vi "Start Plugin.vi"(8 "error in (no error)":errorcluster, 11 "Plugin in":refnum<class "Plugin.lvclass">) -> (0 "error out":errorcluster, 3 "Plugin out":refnum<class "Plugin.lvclass">)   [LabVIEW 2019, in "DSF Core.lvlib" / "Plugin.lvclass"]
uses:
  Plugin.lvclass
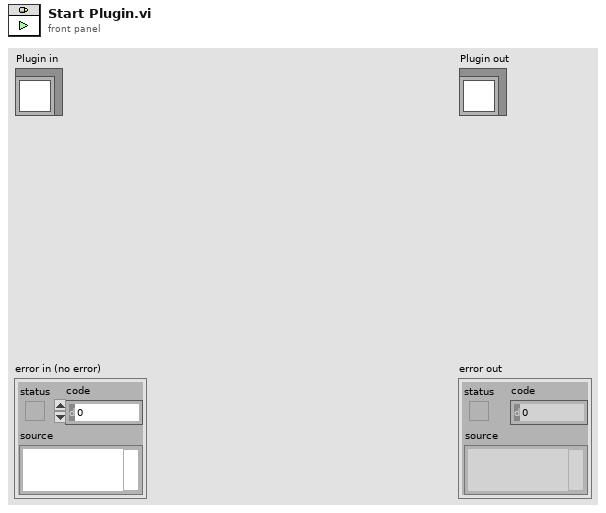
[diagram p1: front panel]
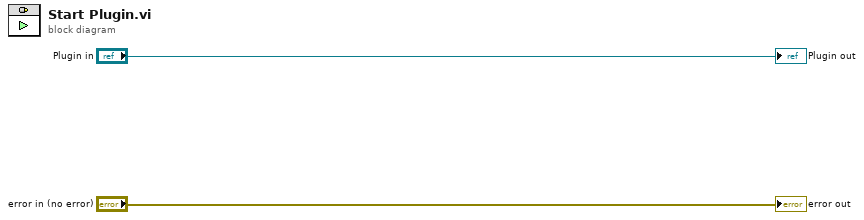
[diagram p0: block diagram]
diagram:
  "error out" <- "error in (no error)"
  "Plugin out" <- "Plugin in"
